vi "Port_Names.vi"() -> ()   [LabVIEW 2017]
uses:
  Anemometry/Anemometry Sub Vis/Controls/ok_button.ctl
  <vilib>/Instr/_visa.llb/VISA Find Search Mode.ctl
  <resource>/objmgr/daqmx.rc
panel:
  out "Dev Numbers":T1(array[cluster])
  out "return count":u32
  out "return count 2":u32
  out "List of Port Names":string[](array[string])
  out "Message":string
  out "List of Canonical Names":string[](array[string])
  in  "OK":T2
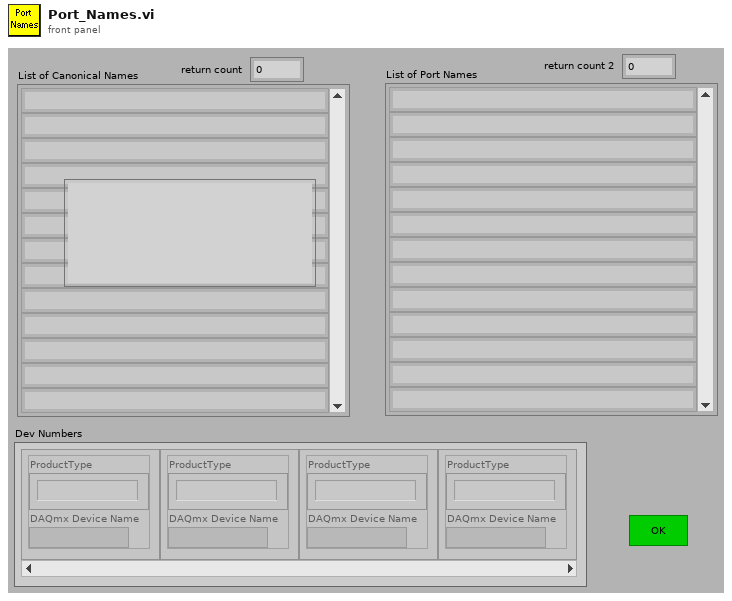
[diagram p1: front panel]
types:
  T1 = cluster{"ProductType":string, "DAQmx Device Name":tag}[]
  T2 = typedef "ok_button.ctl" = bool
  T3 = cluster{"ProductType":string, "DAQmx Device Name":tag}
  T4 = typedef "VISA Find Search Mode.ctl" = u32
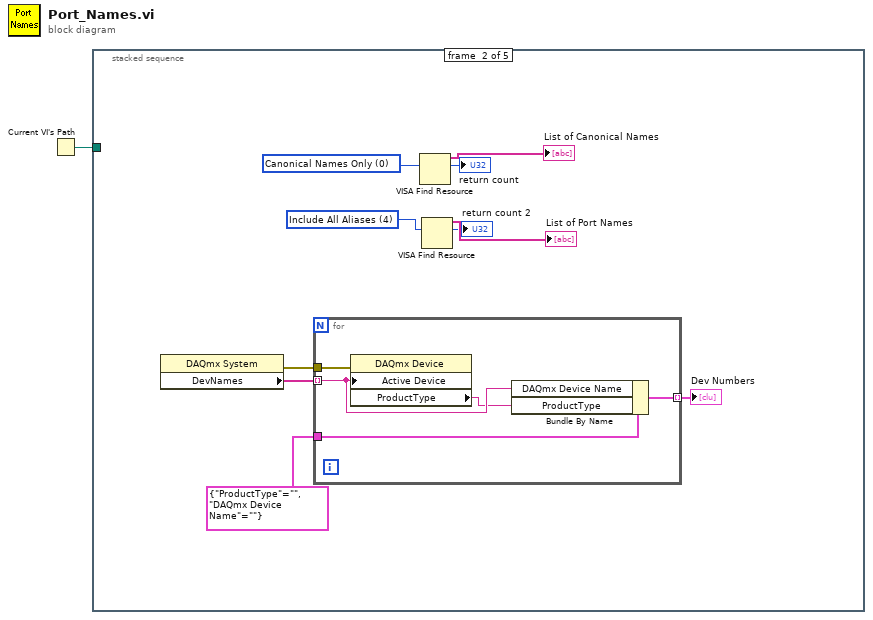
[diagram p0: block diagram]
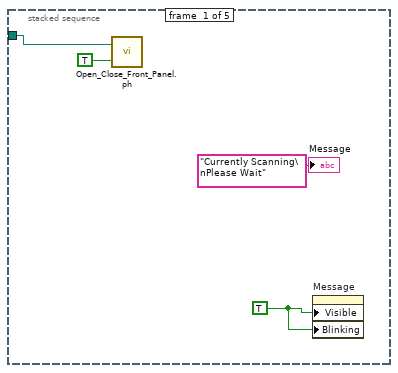
[diagram p2: hidden frame]
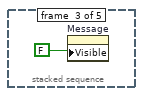
[diagram p3: hidden frame]
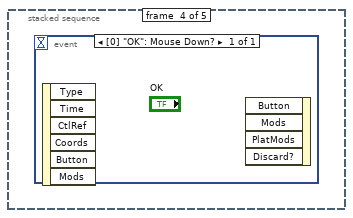
[diagram p4: hidden frame]
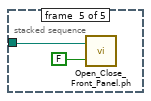
[diagram p5: hidden frame]
diagram:
  n1 = Current VI's Path() -> (path=w1:path)
  n2 = stacked-sequence {
    tunnel: w1 -> [w3 _ _ _ w22]
    frame #0 {
      w2 = TRUE ("Visible")
      n3 = call "Open_Close_Front_Panel.ph.vi"("Front Panel Window:Open"=TRUE, "VI path"=w3) -> ()  [unwired: 2 out]
      n4 = property on="Message" class="Str"("Visible"=w2, "Blinking"=w2) -> ()  [unwired: 2 in, 2 out]
      "Message" <- "Currently Scanning\nPlease Wait" ("Message")
    }
    frame #1 {
      w12 = T4 4 items=["Canonical Names Only"=0, "Aliases Only"=1, "Include Matching Aliases"=2, "Include All Aliases"=4] ("Search Mode")
      w14 = T4 0 items=["Canonical Names Only"=0, "Aliases Only"=1, "Include Matching Aliases"=2, "Include All Aliases"=4] ("Search Mode")
      n5 = property class="DAQmx System"() -> (error out=w7:errorcluster, "DevNames"=w6:tag[])  [unwired: 2 in, 1 out]
      n6 = for {
        tunnel: w6 -> [w18] mode=indexing
        tunnel: w7 -> [w20]
        tunnel: T3 {"ProductType"="", "DAQmx Device Name"=""} ("Cluster") -> [w19]
        tunnel: [w16] -> w9 mode=indexing
        n7 = property class="DAQmx Device"(error in=w20, "Active Device"=w18) -> ("ProductType"=w17:string)  [unwired: 1 in, 2 out]
        n8 = Bundle By Name(cluster=w19, "DAQmx Device Name"=w18, "ProductType"=w17) -> (w16:T3)
      }
      "Dev Numbers" <- w9
      n9 = VISA Find Resource(10:w14) -> (2:→"return count":u32, 3:→"List of Canonical Names":string[])  [unwired: 1 in, 2 out]
      n10 = VISA Find Resource(10:w12) -> (2:→"return count 2":u32, 3:→"List of Port Names":string[])  [unwired: 2 in, 1 out]
    }
    frame #2 {
      n11 = property on="Message" class="Str"("Visible"=FALSE) -> ()  [unwired: 2 in, 2 out]
    }
    frame #3 {
      n12 = event shown="[0] \"OK\": Mouse Down?" {
        selector: _ -> [_]
        dyn-events: _ -> [_]
        timeout: _ -> [_]
        event Mouse Down? {
          n13 = event-data() -> ()  [unwired: 7 out]
          n14 = event-data() -> ()  [unwired: 1 in, 5 out]
        }
      }
    }
    frame #4 {
      n15 = call "Open_Close_Front_Panel.ph.vi"("Front Panel Window:Open"=FALSE, "VI path"=w22) -> ()  [unwired: 2 out]
    }
  }
